vi "Validate Connection.vi"(8 "error in (no error)":errorcluster, 11 "Connection String in":string="host=localhost port=5432 dbname = mydb ") -> (0 "error out":errorcluster, 1 "Status":string, 2 "OK?":bool, 3 "Connection String out":string="host=localhost port=5432 dbname = mydb ")   [LabVIEW 2019, in "LV-Data.PGSQL.lvclass"]
uses:
  LV-Data.PGSQL.lvclass
  <vilib>/JDP Science/PostgreSQL Library/Result/PQ Result.lvclass/PQ Result.ctl
  <vilib>/JDP Science/PostgreSQL Library/Connection/Execute Command (string result).vi
  <vilib>/JDP Science/PostgreSQL Library/Result/Get Column String.vi
  <vilib>/JDP Science/PostgreSQL Library/Result/subVIs/PQ DVR Error.vi
  <vilib>/JDP Science/PostgreSQL Library/Connection/Execute Command (Result).vi
  <vilib>/Utility/error.llb/Error Cluster From Error Code.vi
  <vilib>/JDP Science/PostgreSQL Library/Result/Clear.vi
  <vilib>/JDP Science/PostgreSQL Library/Connection/PQ Connection.lvclass
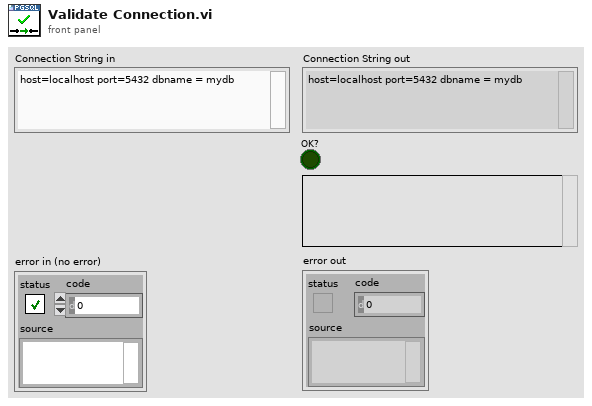
[diagram p1: front panel]
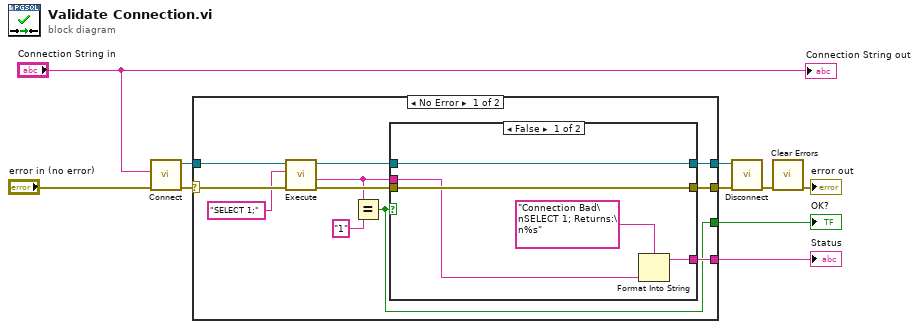
[diagram p0: block diagram]
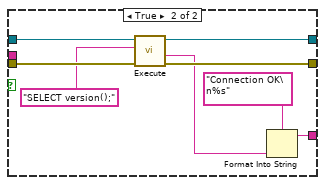
[diagram p2: hidden frame]
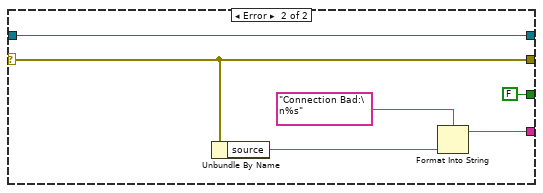
[diagram p3: hidden frame]
diagram:
  n1 = call <vilib>:"Connect.vi"("error in (no error)"="error in (no error)", "Connection Strings"="Connection String in") -> ("error out"=w7:errorcluster, "PQ Connection"=w6:refnum<class "PQ Connection.lvclass">)  [unwired: 8 in]
  n2 = case shown="No Error" w7 {
    selector: w7 -> [w20 w36]
    tunnel: w6 -> [w21 w37]
    tunnel: [w16 w38] -> w8
    tunnel: [w14 w36] -> w9
    tunnel: [w17 w37] -> w2
    tunnel: [w11 FALSE] -> w1
    frame No Error {
      n3 = call-poly <vilib>:"Execute.vi"("error in (no error)"=w20, "SQL"="SELECT 1;", "PQ Connection in"=w21) -> ("error out"=w15:errorcluster, "Result"=w12:string, "PQ Connection out"=w18:refnum<class "PQ Connection.lvclass">)  [unwired: 6 in]
      n4 = Equal?(x=w12, y="1") -> (x = y?=w11:bool)
      n5 = case shown="False" w11 {
        tunnel: w18 -> [w26 w34]
        tunnel: [w26 w33] -> w17
        tunnel: [w23 w31] -> w16
        tunnel: w15 -> [w25 w32]
        tunnel: [w25 w28] -> w14
        tunnel: w12 -> [w22 _]
        frame False {
          n6 = Format Into String(format string="Connection Bad\nSELECT 1; Returns:\n%s", w22) -> (resulting string=w23:string)  [unwired: 2 in, 1 out]
        }
        frame True {
          n7 = call-poly <vilib>:"Execute.vi"("error in (no error)"=w32, "SQL"="SELECT version();", "PQ Connection in"=w34) -> ("error out"=w28:errorcluster, "Result"=w27:string, "PQ Connection out"=w33:refnum<class "PQ Connection.lvclass">)  [unwired: 6 in]
          n8 = Format Into String(format string="Connection OK\n%s", w27) -> (resulting string=w31:string)  [unwired: 2 in, 1 out]
        }
      }
    }
    frame Error {
      n9 = Unbundle By Name(w36) -> ("source"=w39:string)
      n10 = Format Into String(format string="Connection Bad:\n%s", w39) -> (resulting string=w38:string)  [unwired: 2 in, 1 out]
    }
  }
  "Status" <- w8
  "OK?" <- w1
  n11 = call <vilib>:"Disconnect.vi"("error in (no error)"=w9, "PQ Connection in"=w2) -> ("error out"=w10:errorcluster)  [unwired: 9 in]
  n12 = call <vilib>:"Clear Errors.vi"("error in (no error)"=w10) -> ("error out"=→"error out":errorcluster)  [unwired: 5 in, 1 out]
  "Connection String out" <- "Connection String in"
